vi "Handle Error.vi"(5 "Clear Error?":bool=TRUE, 6 "base path":path, 7 "Command":T1=enum."Handle", 8 "error in (no error)":errorcluster, 9 "Classification":T2=enum."Non-Critical", 10 "Section of Code":string, 11 "Test Name":string) -> (0 "error out":errorcluster, 2 "Critical Error":bool, 3 "Non-Critical Error":bool)   [LabVIEW 2024]
doc: "This subVI operates as a modular error handler that can be used multiple times throughout your code.\nWhen initialised it writes a header entry to the error log with the test name and start time.\nWhen handling errors all classification of errors are logged, but warnings are handled without notification to the external system. Critical and non-critical errors are linked to Boolean outputs that can be used to shutdown the system safely or simply inform the user.\nCustom error codes can be handled, by specifying a non-empty array for Error Codes causes the error to be handled only if it matches on of the custom error codes. In this mode, warnings are handled the same as errors.\n\nAuthor: D Keeling\nDate 20/05/2012\nVersion: 1.0"
uses:
  Controls/Error Classification.ctl
  Controls/Error Command.ctl
panel:
  in  "User-Defined Error Codes":i32[](array[numeric]) caption="Error Codes"
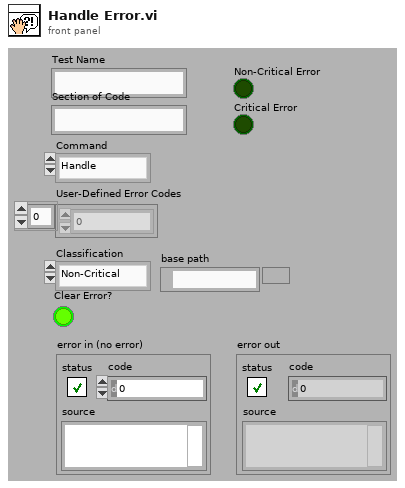
[diagram p1: front panel]
types:
  T1 = typedef "Error Command.ctl" = enum16{"Initialisation", "Handle", "Close"}
  T2 = typedef "Error Classification.ctl" = enum16{"Warning", "Non-Critical", "Critical"}
  T3 = enum16{"open", "replace", "create", "open or create", "replace or create", "replace or create with confirmation"}
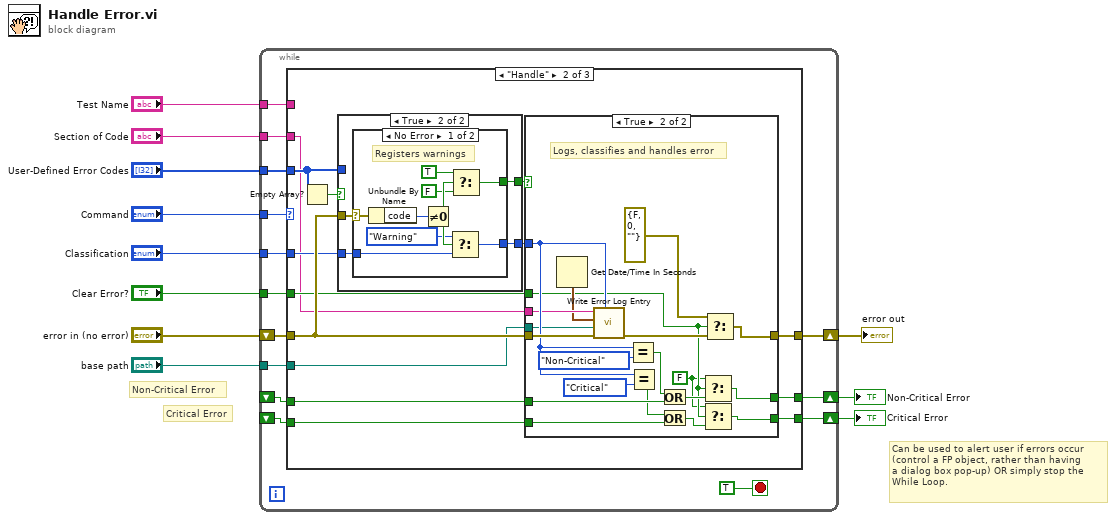
[diagram p0: block diagram]
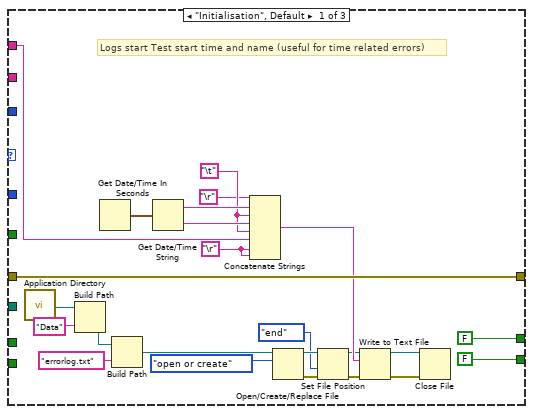
[diagram p2: hidden frame]
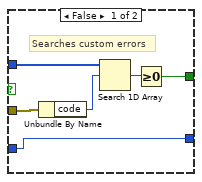
[diagram p4: hidden frame]
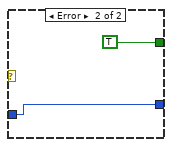
[diagram p5: hidden frame]
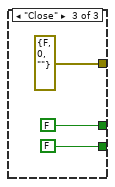
[diagram p6: hidden frame]
diagram:
  # "Can be used to alert user if errors occur\n(control a FP object, rather than having\na dialog box pop-up) OR simply stop the\nWhile Loop."
  # "Critical Error"
  # "Non-Critical Error"
  n1 = while {
    tunnel: "Command" -> [w24]
    shift-right: [w23] -> w5
    shift-left: _ -> [w22]
    shift-right: [w21] -> w4
    shift-left: _ -> [w20]
    shift-right: [w17] -> w8
    shift-left: "error in (no error)" -> [w19]
    tunnel: "User-Defined Error Codes" -> [w18]
    tunnel: "Classification" -> [w16]
    tunnel: "Clear Error?" -> [w15]
    tunnel: "Test Name" -> [w14]
    tunnel: "Section of Code" -> [w13]
    tunnel: "base path" -> [w12]
    stop <- TRUE stop-if-true
    n2 = case shown="\"Handle\"" w24 {
      tunnel: [FALSE ("Session Error") w54 FALSE ("Session Error")] -> w23
      tunnel: w22 -> [_ w57 _]
      tunnel: [FALSE ("System Error") w55 FALSE ("System Error")] -> w21
      tunnel: w20 -> [_ w56 _]
      tunnel: w19 -> [w47 w60 _]
      tunnel: w18 -> [_ w62 _]
      tunnel: [w47 w59 errorcluster {"status"=FALSE, "code"=0, "source"=""} ("error out")] -> w17
      tunnel: w16 -> [_ w53 _]
      tunnel: w15 -> [_ w58 _]
      tunnel: w14 -> [w34 _ _]
      tunnel: w13 -> [_ w51 _]
      tunnel: w12 -> [_ w50 _]
      frame "Initialisation", Default {
        w27 = "\r"
        w35 = "\t"
        # "Logs start Test start time and name (useful for time related errors)"
        n3 = call <vilib>:"Application Directory.vi"() -> ("Application Directory"=w41:path)
        n4 = Build Path(base path=w41, name or relative path="Data") -> (appended path=w43:path)
        n5 = Get Date/Time In Seconds() -> (seconds since 1Jan1904=w36:timestamp)
        n6 = Build Path(base path=w43, name or relative path="errorlog.txt") -> (appended path=w46:path)
        n7 = Get Date/Time String(seconds (now)=w36) -> (date string=w37:string, time string=w38:string)  [unwired: 2 in]
        n8 = Concatenate Strings("\r", w37, w35, w38, w35, w34, w27, w27) -> (w33:string)
        n9 = Open/Create/Replace File(file path (use dialog)=w46, operation (0:open)=T3."open or create") -> (refnum out=w32:refnum<file>, error out=w30:errorcluster)  [unwired: 4 in, 1 out]
        n10 = Set File Position(refnum=w32, from (0:start)=enum16{"start", "end", "current"}."end", error in=w30) -> (refnum out=w29:refnum<file>, error out=w31:errorcluster)  [unwired: 1 in]
        n11 = Write to Text File(file (use dialog)=w29, text=w33, error in=w31) -> (refnum out=w40:refnum<file>, error out=w39:errorcluster)  [unwired: 1 in, 1 out]
        n12 = Close File(refnum=w40, error in=w39) -> ()  [unwired: 2 out]
      }
      frame "Handle" {
        n13 = Empty Array?(array=w62) -> (empty?=w63:bool)
        n14 = case shown="True" w63 {
          tunnel: w60 -> [w92 w96]
          tunnel: w62 -> [w91 _]
          tunnel: [w88 w95] -> w61
          tunnel: w53 -> [w87 w94]
          tunnel: [w87 w93] -> w52
          frame False {
            # "Searches custom errors"
            n15 = Unbundle By Name(w92) -> ("code"=w90:i32)
            n16 = Search 1D Array(1D array=w91, element=w90) -> (index of element=w89:i32)  [unwired: 1 in]
            n17 = Greater Or Equal To 0?(x=w89) -> (x >= 0?=w88:bool)
          }
          frame True {
            n18 = case shown="No Error" w96 {
              selector: w96 -> [w105 _]
              tunnel: [w102 TRUE] -> w95
              tunnel: w94 -> [w98 w106]
              tunnel: [w97 w106] -> w93
              frame No Error {
                # "Registers warnings"
                n19 = Unbundle By Name(w105) -> ("code"=w104:i32)
                n20 = Not Equal To 0?(x=w104) -> (x != 0?=w103:bool)
                n21 = Select(t=Error_Classification."Warning" ("Classification"), s=w103, f=w98) -> (s? t:f=w97:T2)
                n22 = Select(t=TRUE, s=w103, f=FALSE) -> (s? t:f=w102:bool)
              }
              frame Error {
              }
            }
          }
        }
        n23 = case shown="True" w61 {
          tunnel: w51 -> [_ w75]
          tunnel: w60 -> [w66 w86]
          tunnel: [w66 w77] -> w59
          tunnel: w52 -> [_ w80]
          tunnel: w58 -> [_ w70]
          tunnel: w57 -> [w65 w84]
          tunnel: w56 -> [w64 w85]
          tunnel: [w64 w71] -> w55
          tunnel: [w65 w73] -> w54
          tunnel: w50 -> [_ w67]
          frame False {
          }
          frame True {
            w68 = FALSE ("t")
            # "Logs, classifies and handles error"
            n24 = Get Date/Time In Seconds() -> (seconds since 1Jan1904=w74:timestamp)
            n25 = call "Write Error Log Entry.vi"("Classification"=w80, "error in (no error)"=w86, "base path"=w67, "current time"=w74, "Section of System"=w75) -> ("error out"=w78:errorcluster)  [unwired: 6 in]
            n26 = Equal?(x=w80, y=Error_Classification."Non-Critical") -> (x = y?=w81:bool)
            n27 = Equal?(x=w80, y=Error_Classification."Critical") -> (x = y?=w79:bool)
            n28 = Or(x=w81, y=w84) -> (x .or. y?=w72:bool)
            n29 = Or(x=w79, y=w85) -> (x .or. y?=w69:bool)
            n30 = Select(t=w68, s=w70, f=w72) -> (s? t:f=w73:bool)
            n31 = Select(t=w68, s=w70, f=w69) -> (s? t:f=w71:bool)
            n32 = Select(t=errorcluster {"status"=FALSE, "code"=0, "source"=""}, s=w70, f=w78) -> (s? t:f=w77:errorcluster)
          }
        }
      }
      frame "Close" {
      }
    }
  }
  "error out" <- w8
  "Non-Critical Error" <- w5
  "Critical Error" <- w4
